vi "Line-Load Regulation.vi"() -> ()   [LabVIEW 2021]
doc: "Demonstrates how to set up a hardware-timed two-channel nested voltage sweep and display the results in a graph (IV Curve). Use this example to produce the characteristic curves of a FET transistor. It can be easily adapted to test a BJT by performing a current sweep instead of a voltage sweep. This example performs a hardware-timed sweep (with triggers and events) using Sequence source mode."
uses:
  <instrlib>/niDCPower/nidcpower.llb/niDCPower Source Mode.ctl
  <instrlib>/niDCPower/nidcpower.llb/niDCPower Wait For Event - Event.ctl
  <instrlib>/niDCPower/nidcpower.llb/niDCPower Output Function.ctl
  <instrlib>/niDCPower/nidcpower.llb/niDCPower Sequence Attribute Type.ctl
  <instrlib>/niDCPower/nidcpower.llb/niDCPower Sense.ctl
  <instrlib>/niDCPower/nidcpower.llb/niDCPower Create Advanced Sequence Step.vi
  <instrlib>/niDCPower/nidcpower.llb/niDCPower Configure Digital Edge Source Trigger.vi
  <instrlib>/niDCPower/nidcpower.llb/niDCPower Configure Digital Edge Start Trigger.vi
  <instrlib>/niDCPower/nidcpower.llb/niDCPower Configure Digital Edge Sequence Advance Trigger.vi
panel:
  in  "DUT setup time (s)":dbl=1.0
  in  "Sweep type":u16(ring)=1 items=["Linear", "Logarithmic"]
  in  "Source device max. current (A)":dbl=25.0
  in  "Source values (V)":dbl[](array[numeric])=[5.0, 10.0, 15.0, 20.0]
  in  "Timeout (s)":dbl=30.0 format="%.3p"
  in  "Load device name":refnum<k15>="PXI2Slot4"
  in  "Load device source delay (s)":dbl=0.1
  in  "Source device source delay (s)":dbl=0.1
  in  "Load device voltage limit (V)":dbl=5.0
  in  "Source device max. power (W)":dbl=300.0
  in  "Load device channel":string="0"
  in  "Source device channel":string="0"
  out "Current (Amps) vs Voltage (Volts)":T1(graph)
  in  "Points or Points/Decade":i32=10 min=1
  in  "Current load level stop":dbl=2.5 min=0.0 step=0.1
  in  "Current load level start":dbl=0.1 min=0.0 step=0.1
  in  "Source device name":refnum<k15>="PXI2Slot2"
  # "Source Config"
  # "Load config"
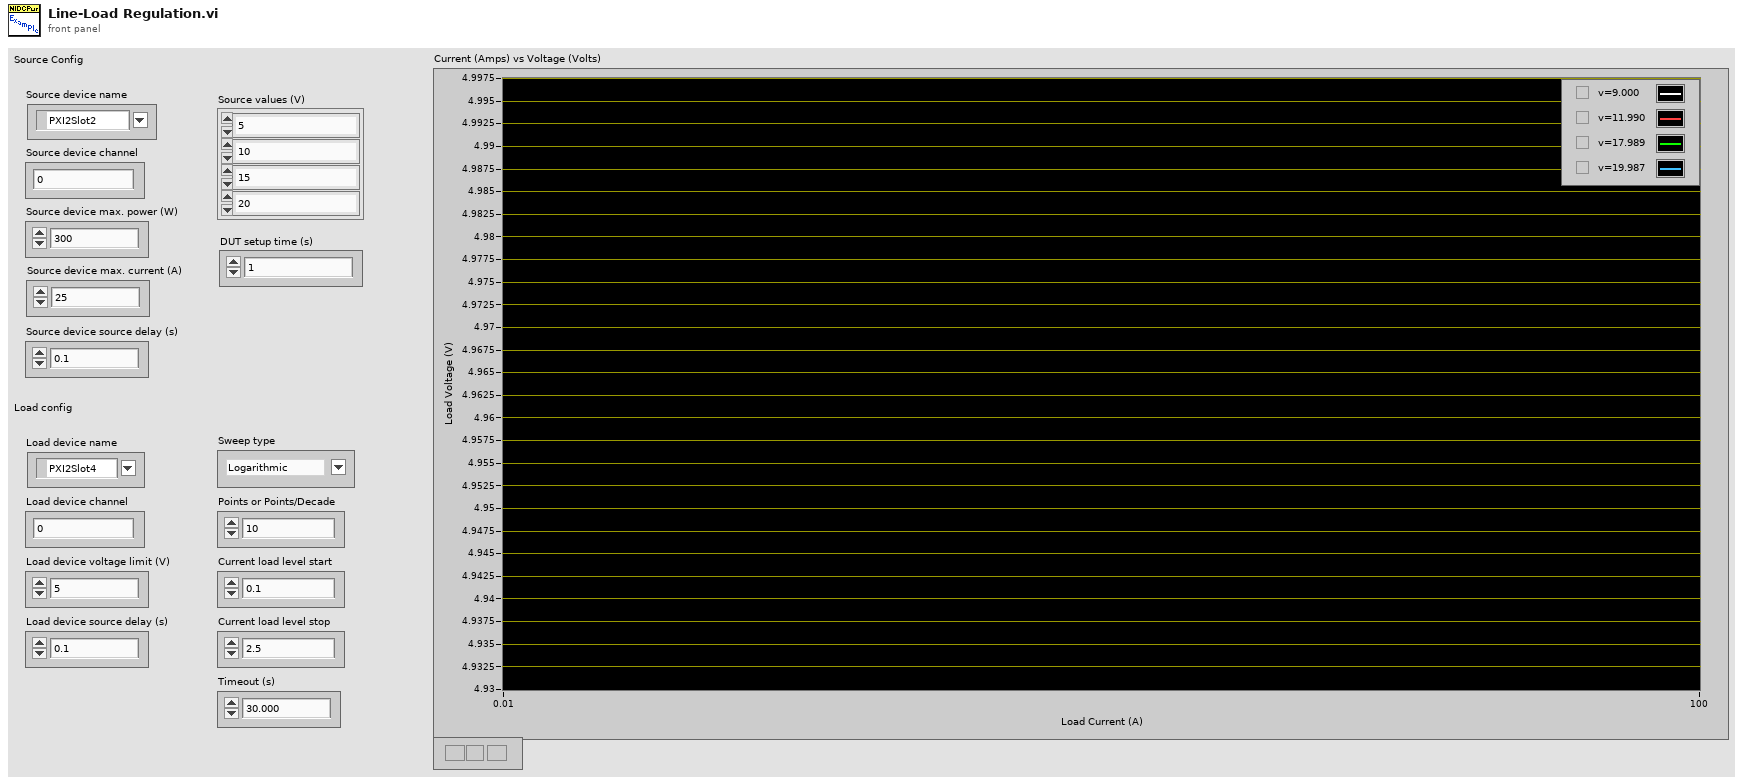
[diagram p1: front panel]
types:
  T1 = cluster{"voltage measurements":dbl[], "current measurements":dbl[]}[]
  T2 = typedef "niDCPower Wait For Event - Event.ctl" = i32
  T3 = typedef "niDCPower Source Mode.ctl" = i32
  T4 = typedef "niDCPower Sense.ctl" = i32
  T5 = typedef "niDCPower Sequence Attribute Type.ctl" = i32
  T6 = typedef "niDCPower Output Function.ctl" = i32
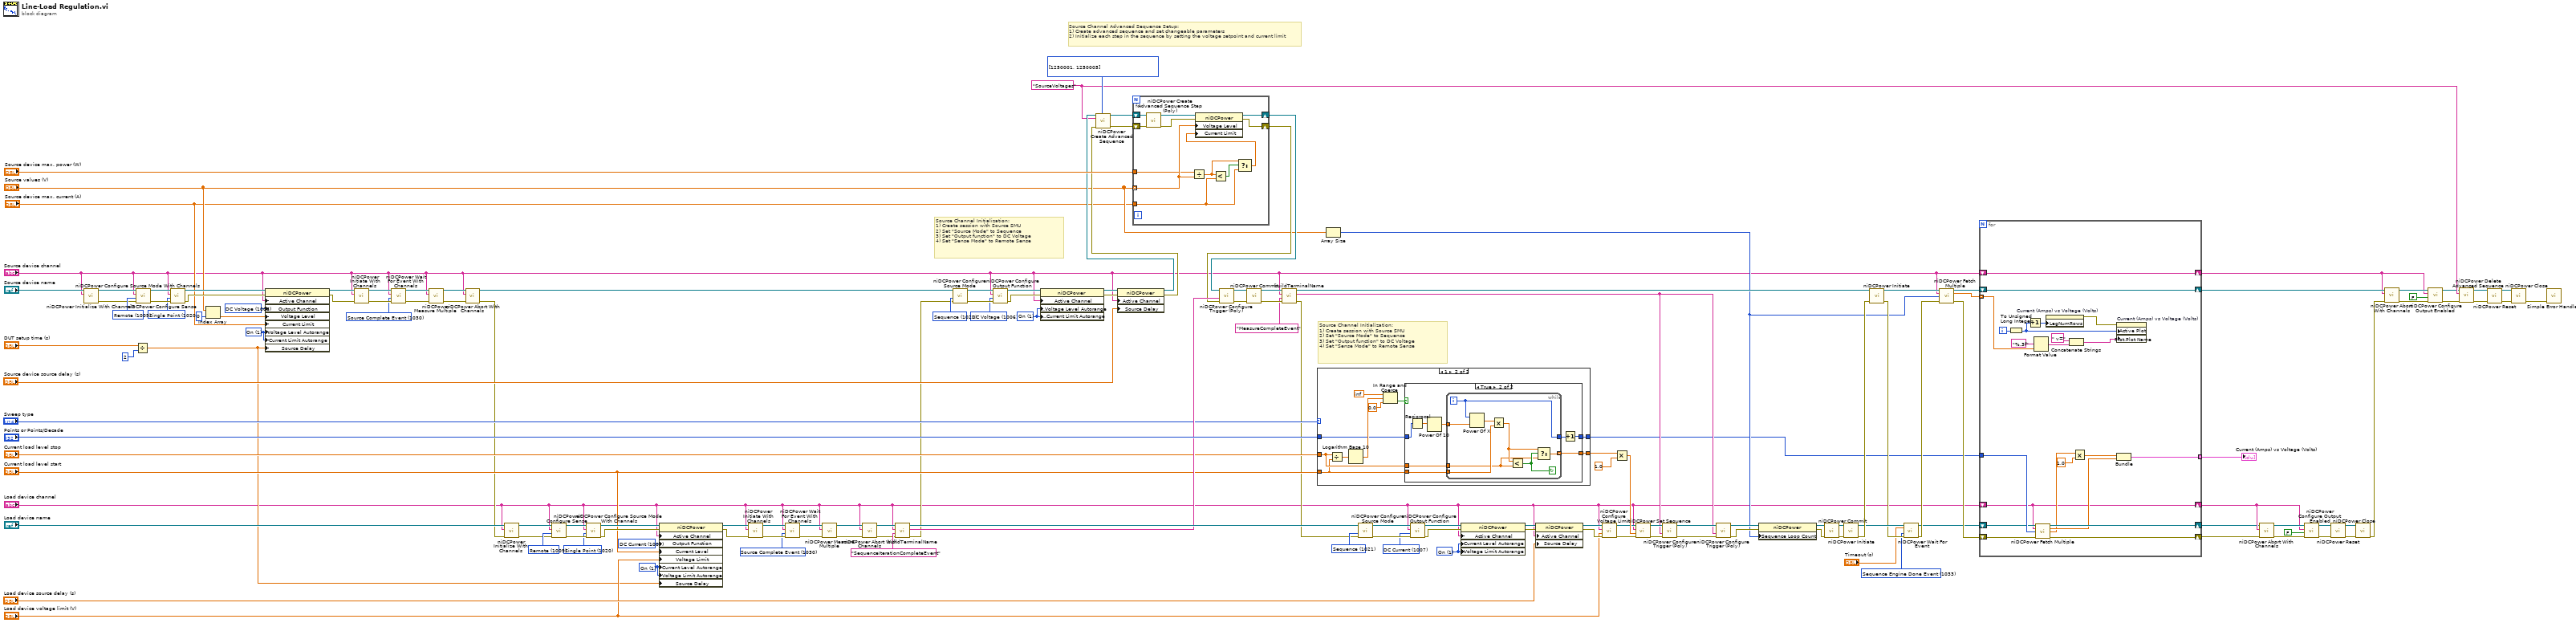
[diagram p0: block diagram]
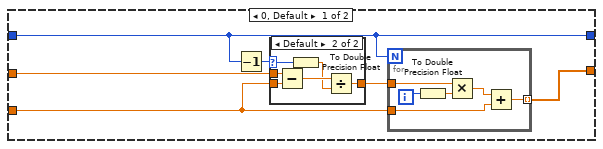
[diagram p2: hidden frame]
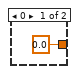
[diagram p3: hidden frame]
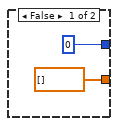
[diagram p4: hidden frame]
diagram:
  w43 = T2 1030 items=["Source Complete Event"=1030, "Measure Complete Event"=1031, "Sequence Iteration Complete Event"=1032, "Sequence Engine Done Event"=1033, "Pulse Complete Event"=1051, "Ready For Pulse Trigger Event"=1052] ("event")
  w48 = 1 items=["Off", "On"] ("Source:DC Current:Current Level Autorange")
  w49 = 1006 items=["DC Voltage"=1006, "DC Current"=1007, "Pulse Voltage"=1049, "Pulse Current"=1050] ("Source:Output Function")
  w50 = T3 1020 items=["Single Point"=1020, "Sequence"=1021] ("source mode")
  w55 = T4 1009 items=["Local"=1008, "Remote"=1009] ("sense")
  w58 = T2 1030 items=["Source Complete Event"=1030, "Measure Complete Event"=1031, "Sequence Iteration Complete Event"=1032, "Sequence Engine Done Event"=1033, "Pulse Complete Event"=1051, "Ready For Pulse Trigger Event"=1052] ("event")
  w63 = 1 items=["Off", "On"] ("Source:DC Current:Current Level Autorange")
  w66 = 1007 items=["DC Voltage"=1006, "DC Current"=1007, "Pulse Voltage"=1049, "Pulse Current"=1050] ("Source:Output Function")
  w69 = T3 1020 items=["Single Point"=1020, "Sequence"=1021] ("source mode")
  w81 = T4 1009 items=["Local"=1008, "Remote"=1009] ("sense")
  w97 = T5[] [1250001, 1250005] items=["Source -> Output Function"=1150008, "Source -> Output Enabled"=1250006, "Source -> Output Resistance"=1150061, "Source -> Transient Response"=1150062, "Source -> Custom Transient Response -> Voltage Gain Bandwidth"=1150067, "Source -> Custom Transient Response -> Voltage Compensation Frequency"=1150068, "Source -> Custom Transient Response -> Voltage Pole-Zero Ratio"=1150069, "Source -> Custom Transient Response -> Current Gain Bandwidth"=1150070, "Source -> Custom Transient Response -> Current Compensation Frequency"=1150071, "Source -> Custom Transient Response -> Current Pole-Zero Ratio"=1150072, "Source -> DC Voltage -> Voltage Level"=1250001, "Source -> DC Voltage -> Voltage Level Range"=1150005, "Source -> DC Voltage -> Current Limit"=1250005, "Source -> DC Voltage -> Current Limit High"=1150187, "Source -> DC Voltage -> Current Limit Low"=1150188, "Source -> DC Voltage -> Current Limit Range"=1150004, "Source -> DC Current -> Current Level"=1150009, "Source -> DC Current -> Current Level Range"=1150011, "Source -> DC Current -> Voltage Limit"=1150010, "Source -> DC Current -> Voltage Limit High"=1150185, "Source -> DC Current -> Voltage Limit Low"=1150186, "Source -> DC Current -> Voltage Limit Range"=1150012, "Source -> Pulse Voltage -> Pulse Voltage Level"=1150080, "Source -> Pulse Voltage -> Pulse Bias Voltage Level"=1150082, "Source -> Pulse Voltage -> Pulse Voltage Level Range"=1150084, "Source -> Pulse Voltage -> Pulse Current Limit"=1150081, "Source -> Pulse Voltage -> Pulse Current Limit High"=1150193, "Source -> Pulse Voltage -> Pulse Current Limit Low"=1150194, "Source -> Pulse Voltage -> Pulse Bias Current Limit"=1150083, "Source -> Pulse Voltage -> Pulse Bias Current Limit High"=1150195, "Source -> Pulse Voltage -> Pulse Bias Current Limit Low"=1150196, "Source -> Pulse Voltage -> Pulse Current Limit Range"=1150085, "Source -> Pulse Current -> Pulse Current Level"=1150086, "Source -> Pulse Current -> Pulse Bias Current Level"=1150088, "Source -> Pulse Current -> Pulse Current Level Range"=1150090, "Source -> Pulse Current -> Pulse Voltage Limit"=1150087, "Source -> Pulse Current -> Pulse Voltage Limit High"=1150189, "Source -> Pulse Current -> Pulse Voltage Limit Low"=1150190, "Source -> Pulse Current -> Pulse Bias Voltage Limit"=1150089, "Source -> Pulse Current -> Pulse Bias Voltage Limit High"=1150191, "Source -> Pulse Current -> Pulse Bias Voltage Limit Low"=1150192, "Source -> Pulse Current -> Pulse Voltage Limit Range"=1150091, "Source -> Advanced -> Source Delay"=1150051, "Source -> Advanced -> Pulse Bias Delay"=1150092, "Source -> Advanced -> Pulse On Time"=1150093, "Source -> Advanced -> Pulse Off Time"=1150094, "Source -> Advanced -> OVP Enabled"=1250002, "Source -> Advanced -> OVP Limit"=1250003, "Source -> Advanced -> Compliance Limit Symmetry"=1150184, "Source -> Advanced -> Sequence Step Delta Time"=1150198, "Measurement -> Sense"=1150013, "Measurement -> Aperture Time"=1150058, "Measurement -> Measure Record Length"=1150063, "Measurement -> Advanced -> DC Noise Rejection"=1150066, "Measurement -> Autorange"=1150244, "Measurement -> Advanced -> Autorange Behavior"=1150245, "Measurement -> Advanced -> Autorange Aperture Time Mode"=1150246, "Measurement -> Advanced -> Autorange Minimum Aperture Time"=1150247, "Measurement -> Advanced -> Autorange Minimum Aperture Time Units"=1150248, "Measurement -> Advanced -> Autorange Minimum Current Range"=1150255, "Measurement -> Advanced -> Autorange Minimum Voltage Range"=1150256, "Measurement -> Advanced -> Autorange Threshold Mode"=1150257, "Measurement -> Advanced -> Autorange Maximum Delay After Range Change"=1150322, "LCR -> Instrument Mode"=1150208, "LCR -> LCR Stimulus Function"=1150209, "LCR -> LCR Frequency"=1150210, "LCR -> LCR Voltage Amplitude"=1150211, "LCR -> LCR Current Amplitude"=1150212, "LCR -> LCR DC Bias Source"=1150213, "LCR -> LCR DC Bias Voltage Level"=1150214, "LCR -> LCR DC Bias Current Level"=1150215, "LCR -> LCR Impedance Autorange"=1150216, "LCR -> LCR Impedance Range"=1150217, "LCR -> LCR Measurement Time"=1150218, "LCR -> LCR Custom Measurement Time"=1150258, "LCR -> LCR Source Delay Mode"=1150315, "LCR -> Compensation -> Open -> Enabled"=1150220, "LCR -> Compensation -> Open -> Conductance"=1150261, "LCR -> Compensation -> Open -> Susceptance"=1150262, "LCR -> Compensation -> Short -> Enabled"=1150221, "LCR -> Compensation -> Short -> Resistance"=1150263, "LCR -> Compensation -> Short -> Reactance"=1150264, "LCR -> Compensation -> Load -> Enabled"=1150222, "LCR -> Compensation -> Load -> Measured Resistance"=1150268, "LCR -> Compensation -> Load -> Measured Reactance"=1150269, "LCR -> Compensation -> Load -> Actual Resistance"=1150270, "LCR -> Compensation -> Load -> Actual Reactance"=1150271] ("advanced sequence properties")
  w87 = "SourceVoltages" ("sequence name")
  w104 = T6 1007 items=["DC Voltage"=1006, "DC Current"=1007, "Pulse Voltage"=1049, "Pulse Current"=1050] ("output function")
  w105 = T6 1006 items=["DC Voltage"=1006, "DC Current"=1007, "Pulse Voltage"=1049, "Pulse Current"=1050] ("output function")
  w121 = T2 1033 items=["Source Complete Event"=1030, "Measure Complete Event"=1031, "Sequence Iteration Complete Event"=1032, "Sequence Engine Done Event"=1033] ("event")
  w139 = T3 1021 items=["Single Point"=1020, "Sequence"=1021] ("source mode")
  w142 = T3 1021 items=["Single Point"=1020, "Sequence"=1021] ("source mode")
  w151 = 1 items=["Off", "On"] ("DC Voltage:Voltage Level Autorange")
  w152 = 1 items=["Off", "On"] ("DC Voltage:Voltage Level Autorange")
  # "Source Channel Initialization:\n1) Create session with Source SMU\n2) Set \"Source Mode\" to Sequence\n3) Set \"Output function\" to DC Voltage\n4) Set \"Sense Mode\" to Remote Sense"
  # "Source Channel Initialization:\n1) Create session with Source SMU\n2) Set \"Source Mode\" to Sequence\n3) Set \"Output function\" to DC Voltage\n4) Set \"Sense Mode\" to Remote Sense"
  # "Source Channel Advanced Sequence Setup:\n1) Create advanced sequence and set changeable parameters\n2) Initialize each step in the sequence by setting the voltage setpoint and current limit"
  n1 = call <instrlib>:"niDCPower Initialize With Channels.vi"("channels"="Source device channel", "resource name"="Source device name") -> ("error out"=w40:errorcluster, "instrument handle out"=w39:refnum<k15>)  [unwired: 3 in, 5 out]
  n2 = Divide(x="DUT setup time (s)", y=2) -> (x/y=w37:dbl)
  n3 = call <instrlib>:"niDCPower Configure Sense.vi"("error in (no error)"=w40, "sense"=w55, "channel name"="Source device channel", "instrument handle"=w39) -> ("error out"=w51:errorcluster, "instrument handle out"=w52:refnum<k15>)  [unwired: 6 in]
  n4 = call <instrlib>:"niDCPower Configure Source Mode With Channels.vi"("error in (no error)"=w51, "source mode"=w50, "channel name"="Source device channel", "instrument handle"=w52) -> ("error out"=w54:errorcluster, "instrument handle out"=w53:refnum<k15>)  [unwired: 6 in]
  n5 = Index Array(array="Source values (V)", index=0) -> (element=w27:dbl)
  n6 = property class="niDCPower"(reference=w53, error in=w54, "Active Channel"="Source device channel", "Output Function"=w49, "Voltage Level"=w27, "Current Limit"="Source device max. current (A)", "Voltage Level Autorange"=w48, "Current Limit Autorange"=w48, "Source Delay"=w37) -> (reference out=w47:refnum<k15>, error out=w46:errorcluster)
  n7 = call <instrlib>:"niDCPower Initiate With Channels.vi"("error in (no error)"=w46, "channel name"="Source device channel", "instrument handle"=w47) -> ("error out"=w44:errorcluster, "instrument handle out"=w45:refnum<k15>)  [unwired: 7 in]
  n8 = call <instrlib>:"niDCPower Wait For Event With Channels.vi"("error in (no error)"=w44, "event"=w43, "channel name"="Source device channel", "instrument handle"=w45) -> ("error out"=w42:errorcluster, "instrument handle out"=w41:refnum<k15>)  [unwired: 6 in]
  n9 = call <instrlib>:"niDCPower Measure Multiple.vi"("error in (no error)"=w42, "channel name"="Source device channel", "instrument handle"=w41) -> ("error out"=w33:errorcluster, "instrument handle out"=w32:refnum<k15>)  [unwired: 5 in, 2 out]
  n10 = call <instrlib>:"niDCPower Abort With Channels.vi"("error in (no error)"=w33, "channel name"="Source device channel", "instrument handle"=w32) -> ("error out"=w23:errorcluster, "instrument handle out"=w24:refnum<k15>)  [unwired: 7 in]
  n11 = call <instrlib>:"niDCPower Initialize With Channels.vi"("error in (no error)"=w23, "channels"="Load device channel", "resource name"="Load device name") -> ("error out"=w71:errorcluster, "instrument handle out"=w70:refnum<k15>)  [unwired: 2 in, 5 out]
  n12 = call <instrlib>:"niDCPower Configure Sense.vi"("error in (no error)"=w71, "sense"=w81, "channel name"="Load device channel", "instrument handle"=w70) -> ("error out"=w72:errorcluster, "instrument handle out"=w73:refnum<k15>)  [unwired: 6 in]
  n13 = call <instrlib>:"niDCPower Configure Source Mode With Channels.vi"("error in (no error)"=w72, "source mode"=w69, "channel name"="Load device channel", "instrument handle"=w73) -> ("error out"=w75:errorcluster, "instrument handle out"=w74:refnum<k15>)  [unwired: 6 in]
  n14 = property class="niDCPower"(reference=w74, error in=w75, "Active Channel"="Load device channel", "Output Function"=w66, "Current Level"="Current load level start", "Voltage Limit"="Load device voltage limit (V)", "Current Level Autorange"=w63, "Voltage Limit Autorange"=w63, "Source Delay"=w37) -> (reference out=w62:refnum<k15>, error out=w61:errorcluster)
  n15 = call <instrlib>:"niDCPower Initiate With Channels.vi"("error in (no error)"=w61, "channel name"="Load device channel", "instrument handle"=w62) -> ("error out"=w59:errorcluster, "instrument handle out"=w60:refnum<k15>)  [unwired: 7 in]
  n16 = call <instrlib>:"niDCPower Wait For Event With Channels.vi"("error in (no error)"=w59, "event"=w58, "channel name"="Load device channel", "instrument handle"=w60) -> ("error out"=w57:errorcluster, "instrument handle out"=w56:refnum<k15>)  [unwired: 6 in]
  n17 = call <instrlib>:"niDCPower Measure Multiple.vi"("error in (no error)"=w57, "channel name"="Load device channel", "instrument handle"=w56) -> ("error out"=w31:errorcluster, "instrument handle out"=w30:refnum<k15>)  [unwired: 5 in, 2 out]
  n18 = call <instrlib>:"niDCPower Abort With Channels.vi"("error in (no error)"=w31, "channel name"="Load device channel", "instrument handle"=w30) -> ("error out"=w22:errorcluster, "instrument handle out"=w29:refnum<k15>)  [unwired: 7 in]
  n19 = call "buildTerminalName.vi"("error in (no error)"=w22, "Local Terminal Name"="SequenceIterationCompleteEvent", "Channel Name"="Load device channel", "session handle"=w29) -> ("error IO"=w21:errorcluster, "Fully Qualified Terminal Name"=w109:string, "session handle 2"=w110:refnum<k15>)  [unwired: 5 out]
  n20 = call <instrlib>:"niDCPower Configure Source Mode.vi"("error in (no error)"=w21, "source mode"=w142, "instrument handle"=w24) -> ("error out"=w144:errorcluster, "instrument handle out"=w143:refnum<k15>)  [unwired: 7 out]
  n21 = call <instrlib>:"niDCPower Configure Output Function.vi"("error in (no error)"=w144, "output function"=w105, "channel name"="Source device channel", "instrument handle"=w143) -> ("error out"=w34:errorcluster, "instrument handle out"=w35:refnum<k15>)  [unwired: 6 out]
  n22 = property class="niDCPower"(reference=w35, error in=w34, "Active Channel"="Source device channel", "Source:DC Voltage:Voltage Level Autorange"=w152, "Source:DC Voltage:Current Limit Autorange"=w152) -> (reference out=w136:refnum<k15>, error out=w135:errorcluster)
  n23 = property class="niDCPower"(reference=w136, error in=w135, "Active Channel"="Source device channel", "Source Delay"="Source device source delay (s)") -> (reference out=w95:refnum<k15>, error out=w94:errorcluster)
  n24 = call <instrlib>:"niDCPower Create Advanced Sequence.vi"("instrument handle"=w95, "sequence name"=w87, "advanced sequence properties"=w97, "error in (no error)"=w94) -> ("instrument handle out"=w99:refnum<k15>, "error out"=w98:errorcluster)  [unwired: 10 in]
  n25 = for {
    shift-right: [w162] -> w93
    shift-left: w98 -> [w165]
    shift-right: [w161] -> w92
    shift-left: w99 -> [w160]
    tunnel: "Source device max. power (W)" -> [w158]
    tunnel: "Source values (V)" -> [w159] mode=indexing
    tunnel: "Source device max. current (A)" -> [w156]
    n26 = call-poly <instrlib>:"niDCPower Create Advanced Sequence Step (Poly).vi"("error in (no error)"=w165, "instrument handle"=w160) -> ("error out"=w163:errorcluster, "instrument handle out"=w164:refnum<k15>)  [unwired: 8 in]
    n27 = Divide(x=w158, y=w159) -> (x/y=w155:dbl)
    n28 = Less?(x=w155, y=w156) -> (x < y?=w157:bool)
    n29 = Select(t=w155, s=w157, f=w156) -> (s? t:f=w154:dbl)
    n30 = property class="niDCPower"(reference=w164, error in=w163, "Voltage Level"=w159, "Current Limit"=w154) -> (reference out=w161:refnum<k15>, error out=w162:errorcluster)
  }
  n31 = call-poly <instrlib>:"niDCPower Configure Trigger (Poly).vi"("error in (no error)"=w93, "input terminal"=w109, "instrument handle"=w92) -> ("error out"=w148:errorcluster, "instrument handle out"=w147:refnum<k15>)  [unwired: 1 in, 6 out]
  n32 = call <instrlib>:"niDCPower Commit.vi"("error in (no error)"=w148, "instrument handle"=w147) -> ("error out"=w115:errorcluster, "instrument handle out"=w114:refnum<k15>)  [unwired: 8 out]
  n33 = call "buildTerminalName.vi"("error in (no error)"=w115, "Local Terminal Name"="MeasureCompleteEvent" ("Channel Name"), "Channel Name"="Source device channel", "session handle"=w114) -> ("error IO"=w20:errorcluster, "Fully Qualified Terminal Name"=w111:string, "session handle 2"=w113:refnum<k15>)  [unwired: 5 out]
  n34 = case shown="1" "Sweep type" {
    tunnel: "Points or Points/Decade" -> [w166 w185]
    tunnel: [w169 w189] -> w102
    tunnel: "Current load level start" -> [w168 w186]
    tunnel: "Current load level stop" -> [w167 w193]
    tunnel: [w166 w190] -> w78
    frame 0, Default {
      n35 = Decrement(x=w166) -> (x-1=w171:i32)
      n36 = case shown="Default" w171 {
        selector: w171 -> [_ w179]
        tunnel: w167 -> [_ w184]
        tunnel: w168 -> [_ w183]
        tunnel: [0.0 w181] -> w170
        frame 0 {
        }
        frame Default {
          n37 = Subtract(x=w184, y=w183) -> (x-y=w182:dbl)
          n38 = To Double Precision Float(number=w179) -> (double precision float=w180:dbl)
          n39 = Divide(x=w182, y=w180) -> (x/y=w181:dbl)
        }
      }
      n40 = for {
        N: w166 -> [_]
        tunnel: w170 -> [w176]
        tunnel: w168 -> [w177]
        tunnel: [w172] -> w169 mode=indexing
        i -> [w175]
        n41 = To Double Precision Float(number=w175) -> (double precision float=w173:dbl)
        n42 = Multiply(x=w176, y=w173) -> (x*y=w174:dbl)
        n43 = Add(x=w174, y=w177) -> (x+y=w172:dbl)
      }
    }
    frame 1 {
      n44 = Divide(x=w193, y=w186) -> (x/y=w194:dbl)
      n45 = Logarithm Base 10(1:w194) -> (0:w191:dbl)
      n46 = In Range and Coerce(upper limit=inf, x=w191, lower limit=0.0) -> (In Range?=w188:bool)  [unwired: 1 out]
      n47 = case shown="True" w188 {
        tunnel: [dbl[] [] w204] -> w189
        tunnel: [0 w197] -> w190
        tunnel: w193 -> [_ w203]
        tunnel: w186 -> [_ w202]
        tunnel: w185 -> [_ w199]
        frame False {
        }
        frame True {
          n48 = Reciprocal(x=w199) -> (1/x=w201:dbl)
          n49 = Power Of 10(x=w201) -> (10^x=w200:dbl)
          n50 = while {
            tunnel: w200 -> [w209]
            tunnel: w202 -> [w212]
            tunnel: [w208] -> w204 mode=indexing
            tunnel: [w210] -> w198
            tunnel: w203 -> [w205]
            i -> [w210]
            stop <- w207 continue-if-true
            n51 = Power Of X(1:w209, 2:w210) -> (0:w211:dbl)
            n52 = Multiply(x=w211, y=w212) -> (x*y=w206:dbl)
            n53 = Less?(x=w206, y=w205) -> (x < y?=w207:bool)
            n54 = Select(t=w206, s=w207, f=w205) -> (s? t:f=w208:dbl)
          }
          n55 = Increment(x=w198) -> (x+1=w197:i32)
        }
      }
    }
  }
  n56 = Array Size(array="Source values (V)") -> (size(s)=w103:i32)
  n57 = call <instrlib>:"niDCPower Configure Source Mode.vi"("error in (no error)"=w20, "source mode"=w139, "instrument handle"=w110) -> ("error out"=w141:errorcluster, "instrument handle out"=w140:refnum<k15>)  [unwired: 7 out]
  n58 = call <instrlib>:"niDCPower Configure Output Function.vi"("error in (no error)"=w141, "output function"=w104, "channel name"="Load device channel", "instrument handle"=w140) -> ("error out"=w67:errorcluster, "instrument handle out"=w68:refnum<k15>)  [unwired: 6 out]
  n59 = property class="niDCPower"(reference=w68, error in=w67, "Active Channel"="Load device channel", "Current Level Autorange"=w151, "Voltage Limit Autorange"=w151) -> (reference out=w133:refnum<k15>, error out=w132:errorcluster)
  n60 = property class="niDCPower"(reference=w133, error in=w132, "Active Channel"="Load device channel", "Source Delay"="Load device source delay (s)") -> (reference out=w85:refnum<k15>, error out=w86:errorcluster)
  n61 = call <instrlib>:"niDCPower Configure Voltage Limit.vi"("error in (no error)"=w86, "voltage limit"="Load device voltage limit (V)", "channel name"="Load device channel", "instrument handle"=w85) -> ("error out"=w83:errorcluster, "instrument handle out"=w84:refnum<k15>)  [unwired: 6 in]
  n62 = Multiply(x=w102, y=1.0) -> (x*y=w101:dbl[])
  n63 = call <instrlib>:"niDCPower Set Sequence.vi"("error in (no error)"=w83, "values"=w101, "channel name"="Load device channel", "instrument handle"=w84) -> ("error out"=w128:errorcluster, "instrument handle out"=w129:refnum<k15>)  [unwired: 1 in, 5 out]
  n64 = call-poly <instrlib>:"niDCPower Configure Trigger (Poly).vi"("error in (no error)"=w128, "input terminal"=w111, "instrument handle"=w129) -> ("error out"=w127:errorcluster, "instrument handle out"=w126:refnum<k15>)  [unwired: 1 in, 6 out]
  n65 = call-poly <instrlib>:"niDCPower Configure Trigger (Poly).vi"("error in (no error)"=w127, "input terminal"=w111, "instrument handle"=w126) -> ("error out"=w118:errorcluster, "instrument handle out"=w119:refnum<k15>)  [unwired: 1 in, 6 out]
  n66 = property class="niDCPower"(reference=w119, error in=w118, "Sequence Loop Count"=w103) -> (reference out=w116:refnum<k15>, error out=w117:errorcluster)
  n67 = call <instrlib>:"niDCPower Commit.vi"("error in (no error)"=w117, "instrument handle"=w116) -> ("error out"=w150:errorcluster, "instrument handle out"=w80:refnum<k15>)  [unwired: 8 out]
  n68 = call <instrlib>:"niDCPower Initiate.vi"("error in (no error)"=w150, "instrument handle"=w80) -> ("error out"=w149:errorcluster, "instrument handle out"=w125:refnum<k15>)  [unwired: 8 out]
  n69 = call <instrlib>:"niDCPower Initiate.vi"("error in (no error)"=w149, "instrument handle"=w113) -> ("error out"=w124:errorcluster, "instrument handle out"=w120:refnum<k15>)  [unwired: 8 out]
  n70 = call <instrlib>:"niDCPower Wait For Event.vi"("timeout (10.0)"="Timeout (s)", "error in (no error)"=w124, "event"=w121, "instrument handle"=w125) -> ("error out"=w123:errorcluster, "instrument handle out"=w122:refnum<k15>)  [unwired: 6 out]
  n71 = call <instrlib>:"niDCPower Fetch Multiple.vi"("instrument handle"=w120, "channel name"="Source device channel", "count (1)"=w103, "error in (no error)"=w123) -> ("instrument handle out"=w17:refnum<k15>, "voltage measurements"=w106:dbl[], "error out"=w138:errorcluster)  [unwired: 1 in, 8 out]
  n72 = for {
    shift-right: [w223] -> w4
    shift-left: w138 -> [w224]
    tunnel: [w222] -> w137 mode=indexing
    tunnel: w106 -> [w226] mode=indexing
    tunnel: w78 -> [w225]
    shift-right: [w221] -> w3
    shift-left: w122 -> [w220]
    shift-right: [w217] -> w16
    shift-left: w17 -> [w217]
    shift-right: [w214] -> w5
    shift-left: "Load device channel" -> [w214]
    shift-right: [w213] -> w2
    shift-left: "Source device channel" -> [w213]
    i -> [w229]
    n73 = To Unsigned Long Integer(number=w229) -> (unsigned 32bit integer=w228:u32)
    n74 = Increment(x=w228) -> (x+1=w227:u32)
    n75 = Format Value(format string="%.3f", value (0)=w226) -> (output string=w232:string)  [unwired: 1 out]
    n76 = call <instrlib>:"niDCPower Fetch Multiple.vi"("instrument handle"=w220, "channel name"=w214, "count (1)"=w225, "error in (no error)"=w224) -> ("instrument handle out"=w221:refnum<k15>, "voltage measurements"=w218:dbl[], "current measurements"=w215:dbl[], "error out"=w223:errorcluster)  [unwired: 1 in, 7 out]
    n77 = property on="Current (Amps) vs Voltage (Volts)" class="XYGraph (strict)"("LegNumRows"=w227) -> (error out=w230:errorcluster)  [unwired: 2 in, 1 out]
    n78 = Concatenate Strings(" v=" ("string"), w232) -> (w231:string)
    n79 = Multiply(x=w215, y=1.0) -> (x*y=w219:dbl[])
    n80 = property on="Current (Amps) vs Voltage (Volts)" class="XYGraph (strict)"(error in=w230, "Active Plot"=w228, "Plot.Plot Name"=w231) -> ()  [unwired: 1 in, 2 out]
    n81 = Bundle(w219, "voltage measurements"=w218) -> (w222:cluster{dbl[], "voltage measurements":dbl[]})  [unwired: 1 out]
  }
  "Current (Amps) vs Voltage (Volts)" <- w137
  n82 = call <instrlib>:"niDCPower Abort With Channels.vi"("error in (no error)"=w4, "channel name"=w5, "instrument handle"=w3) -> ("error out"=w6:errorcluster, "instrument handle out"=w7:refnum<k15>)  [unwired: 7 in]
  n83 = call <instrlib>:"niDCPower Configure Output Enabled.vi"("error in (no error)"=w6, "output enabled"=FALSE, "channel name"=w5, "instrument handle"=w7) -> ("error out"=w8:errorcluster, "instrument handle out"=w9:refnum<k15>)  [unwired: 6 out]
  n84 = call <instrlib>:"niDCPower Reset.vi"("error in (no error)"=w8, "instrument handle"=w9) -> ("error out"=w76:errorcluster, "instrument handle out"=w77:refnum<k15>)  [unwired: 2 in, 6 out]
  n85 = call <instrlib>:"niDCPower Close.vi"("error in (no error)"=w76, "instrument handle"=w77) -> ("error out"=w18:errorcluster)  [unwired: 9 out]
  n86 = call <instrlib>:"niDCPower Abort With Channels.vi"("error in (no error)"=w18, "channel name"=w2, "instrument handle"=w16) -> ("error out"=w15:errorcluster, "instrument handle out"=w14:refnum<k15>)  [unwired: 7 in]
  n87 = call <instrlib>:"niDCPower Configure Output Enabled.vi"("error in (no error)"=w15, "output enabled"=FALSE, "channel name"=w2, "instrument handle"=w14) -> ("error out"=w12:errorcluster, "instrument handle out"=w13:refnum<k15>)  [unwired: 6 in]
  n88 = call <instrlib>:"niDCPower Delete Advanced Sequence.vi"("error in (no error)"=w12, "sequence name"=w87, "instrument handle"=w13) -> ("error out"=w88:errorcluster, "instrument handle out"=w89:refnum<k15>)  [unwired: 7 in]
  n89 = call <instrlib>:"niDCPower Reset.vi"("error in (no error)"=w88, "instrument handle"=w89) -> ("error out"=w90:errorcluster, "instrument handle out"=w91:refnum<k15>)  [unwired: 2 in, 6 out]
  n90 = call <instrlib>:"niDCPower Close.vi"("error in (no error)"=w90, "instrument handle"=w91) -> ("error out"=w1:errorcluster)  [unwired: 9 out]
  n91 = call <vilib>:"Simple Error Handler.vi"("error in (no error)"=w1) -> ()  [unwired: 1 in, 8 out]
